vi "rampStates.vi"(6 "motor2Stop":bool, 7 "endGame?":bool, 9 "buttonsPushed?":bool, 10 "motor1Stop":bool, 11 "stage2Clear?":bool) -> (1 "Current State":T1, 2 "motor2":bool, 3 "motor1":bool)   [LabVIEW 2017]
uses:
  rampStates.ctl
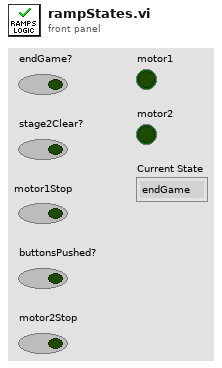
[diagram p1: front panel]
types:
  T1 = typedef "rampStates.ctl" = enum16{"endGame", "finish", "idle", "deploy"}
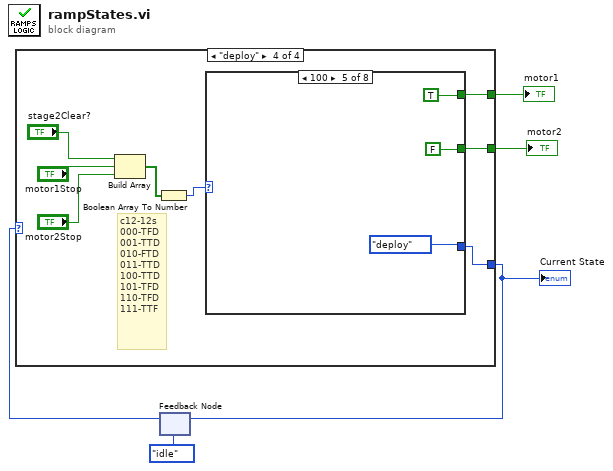
[diagram p0: block diagram]
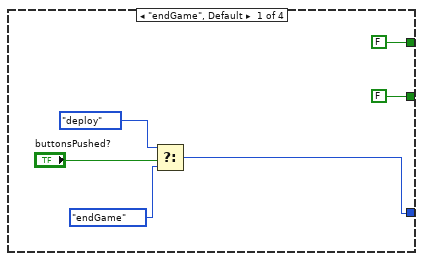
[diagram p2: hidden frame]
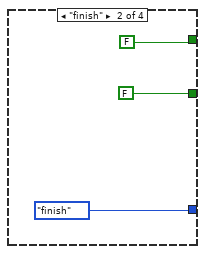
[diagram p3: hidden frame]
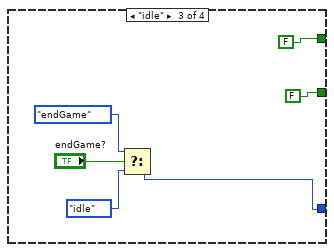
[diagram p4: hidden frame]
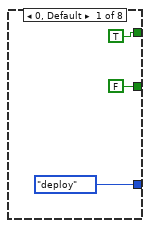
[diagram p5: hidden frame]
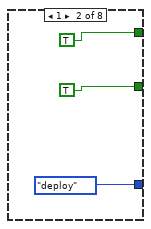
[diagram p6: hidden frame]
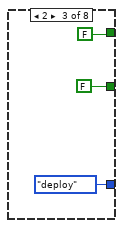
[diagram p7: hidden frame]
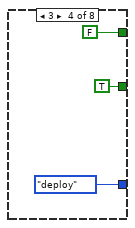
[diagram p8: hidden frame]
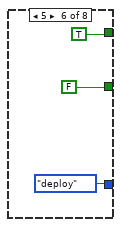
[diagram p9: hidden frame]
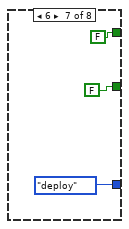
[diagram p10: hidden frame]
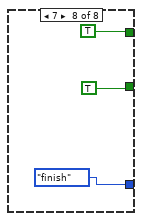
[diagram p11: hidden frame]
diagram:
  n1 = feedback #1(rampStates."idle") -> (w2:T1)
  n2 = case shown="\"deploy\"" w2 {
    tunnel: [w6 rampStates."finish" w17 w26] -> w3
    tunnel: [FALSE FALSE FALSE w24] -> w4
    tunnel: [FALSE FALSE FALSE w25] -> w5
    frame "endGame", Default {
      n3 = Select(t=rampStates."deploy", s="buttonsPushed?", f=rampStates."endGame") -> (s? t:f=w6:T1)
    }
    frame "finish" {
    }
    frame "idle" {
      n4 = Select(t=rampStates."endGame", s="endGame?", f=rampStates."idle") -> (s? t:f=w17:T1)
    }
    frame "deploy" {
      # "c12-12s\n000-TFD\n001-TTD\n010-FTD\n011-TTD\n100-TTD\n101-TFD\n110-TFD\n111-TTF"
      n5 = Build Array("stage2Clear?", "motor1Stop", "motor2Stop") -> (w28:bool[])
      n6 = Boolean Array To Number(Boolean array=w28) -> (number=w27:u32)
      n7 = case shown="100" w27 {
        tunnel: [rampStates."deploy" rampStates."deploy" rampStates."deploy" rampStates."deploy" rampStates."deploy" rampStates."deploy" rampStates."deploy" rampStates."finish"] -> w26
        tunnel: [TRUE TRUE FALSE FALSE TRUE TRUE FALSE TRUE] -> w25
        tunnel: [FALSE TRUE FALSE TRUE FALSE FALSE FALSE TRUE] -> w24
        frame 0, Default {
        }
        frame 1 {
        }
        frame 2 {
        }
        frame 3 {
        }
        frame 4 {
        }
        frame 5 {
        }
        frame 6 {
        }
        frame 7 {
        }
      }
    }
  }
  "motor1" <- w5
  "motor2" <- w4
  "Current State" <- w3
  n8 = feedback-in #1(w3) -> ()
